vi "Generic command handler.vi"(8 "error in (no error)":errorcluster, 10 "Message in":refnum<class "GenericMessage.lvclass">, 11 "AOTF in":refnum<class "AOTF.lvclass">) -> (0 "error out":errorcluster, 2 "command":string, 3 "AOTF out":refnum<class "AOTF.lvclass">)   [LabVIEW 2012, in "AOTF.lvclass"]
doc: "The generic_command_handler processes the command 'generic'. Commands which are not part of the predefined list of commands fall under the 'generic' command for special activity."
uses:
  AOTF.lvclass
  <vilib>/Distrio/Murmex/GenericMessage/GenericMessage.lvclass
  <vilib>/Distrio/Murmex/Murmex/Murmex.lvclass
  Controls/laser line ring.ctl
  AOTF.lvclass/AOTF.ctl
panel:
  # "This method is called when the GENERIC\ntrigger is sent. \n\nOverride this method when your component needs to\nrespond to this trigger. \n\nCall parent for proper implementation"
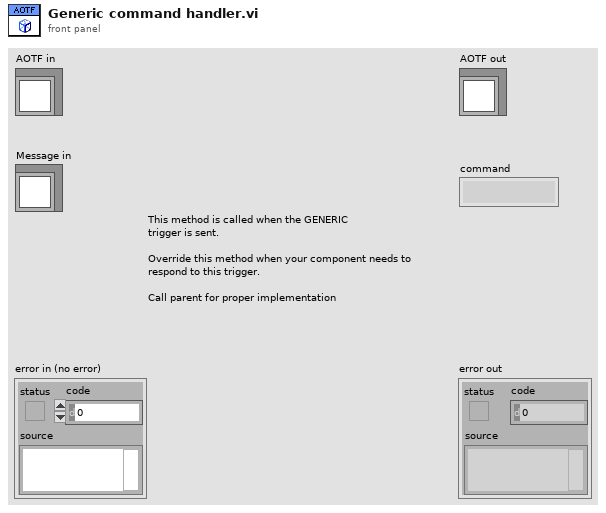
[diagram p1: front panel]
types:
  T1 = typedef "AOTF.lvclass/laser line ring.ctl" = u8
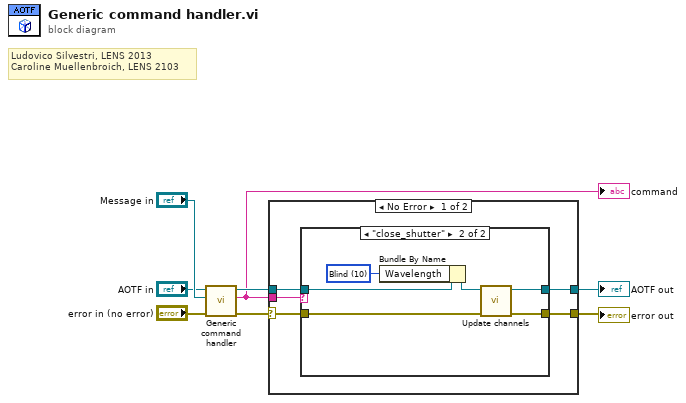
[diagram p0: block diagram]
diagram:
  # "Ludovico Silvestri, LENS 2013\nCaroline Muellenbroich, LENS 2103"
  n1 = call-parent "Generic command handler.vi"("error in (no error)"="error in (no error)", "Message in"="Message in", "Murmex in"="AOTF in") -> ("error out"=w5:errorcluster, "value"=w1:string, "Murmex out"=w2:refnum<class "AOTF.lvclass">)  [unwired: 6 in]
  "command" <- w1
  n2 = case shown="No Error" w5 {
    selector: w5 -> [w9 w23]
    tunnel: [w10 w23] -> w4
    tunnel: [w12 w22] -> w3
    tunnel: w2 -> [w11 w22]
    tunnel: w1 -> [w13 _]
    frame No Error {
      n3 = case shown="\"close_shutter\"" w13 {
        tunnel: [w15 w16] -> w12
        tunnel: w11 -> [w15 w21]
        tunnel: [w14 w18] -> w10
        tunnel: w9 -> [w14 w19]
        frame Default {
        }
        frame "close_shutter" {
          w20 = T1 10 items=["Blind"=10, "405nm"=0, "445nm"=5, "491nm"=1, "515nm"=2, "561nm"=3] ("Settings cluster.Wavelength")
          n4 = Bundle By Name(cluster=w21, "Wavelength"=w20) -> (w17:refnum<class "AOTF.lvclass">)
          n5 = call-dynamic "Update channels.vi"("error in (no error)"=w19, "AOTF in"=w17) -> ("error out"=w18:errorcluster, "AOTF out"=w16:refnum<class "AOTF.lvclass">)  [unwired: 8 in]
        }
      }
    }
    frame Error {
    }
  }
  "error out" <- w4
  "AOTF out" <- w3
